vi "S2C_PCIe7841_Proc_Status.vi"(8 "Error In":errorcluster) -> (0 "Error Out":errorcluster, 3 "Response":string)   [LabVIEW 2015]
uses:
  S2C_PCIe7841_Proc_Globals.vi
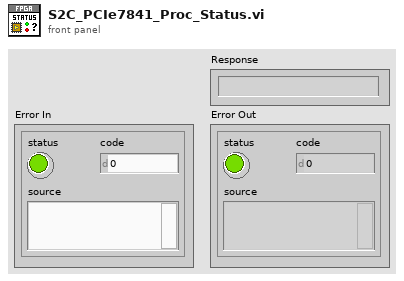
[diagram p1: front panel]
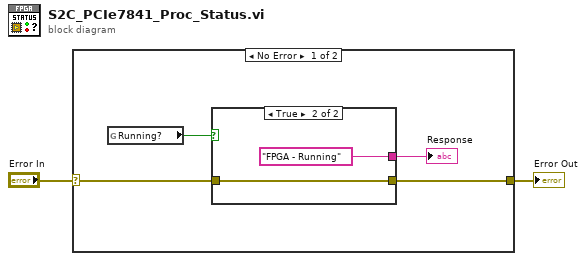
[diagram p0: block diagram]
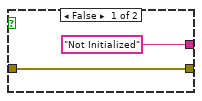
[diagram p2: hidden frame]
diagram:
  n1 = case shown="No Error" "Error In" {
    selector: "Error In" -> [w6 w11]
    tunnel: [w5 w11] -> w1
    frame No Error {
      n2 = global read "S2C_PCIe7841_Proc_Globals.vi" "Running?"() -> (w3:bool)
      n3 = case shown="True" w3 {
        tunnel: w6 -> [w8 w10]
        tunnel: [w8 w10] -> w5
        tunnel: ["Not Initialized" "FPGA - Running" ("f")] -> w4
        frame False {
        }
        frame True {
        }
      }
      "Response" <- w4
    }
    frame Error {
    }
  }
  "Error Out" <- w1
